vi "read write basic.vi"() -> ()   [LabVIEW 2021]
uses:
  <vilib>/Utility/file.llb/Read Delimited Spreadsheet (string).vi
  <vilib>/Utility/file.llb/Write Delimited Spreadsheet (string).vi
panel:
  out "Read Data":cluster{"Temp Data":dbl, "Message":string}[](array[cluster])
  in  "Write Data":cluster{"Temp Data":dbl, "Message":string}[](array[cluster])
  in  "Write and Read data":bool
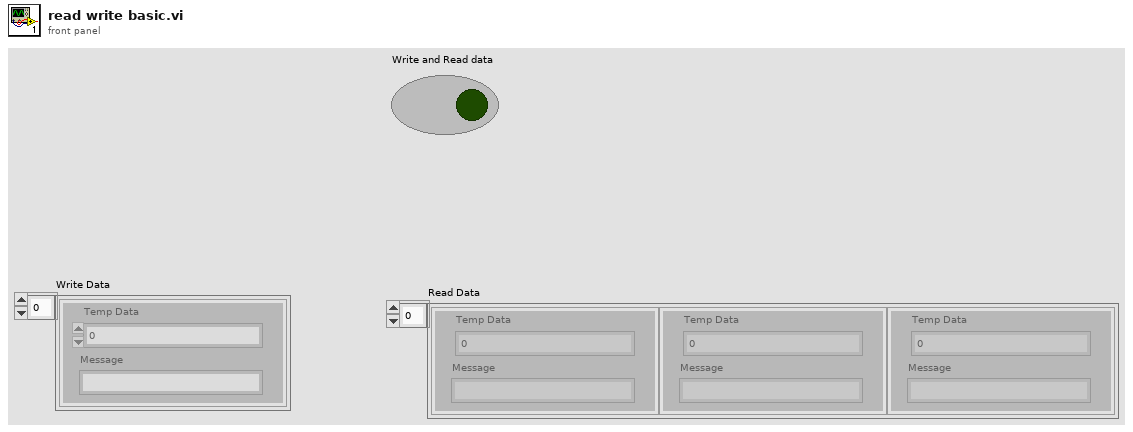
[diagram p1: front panel]
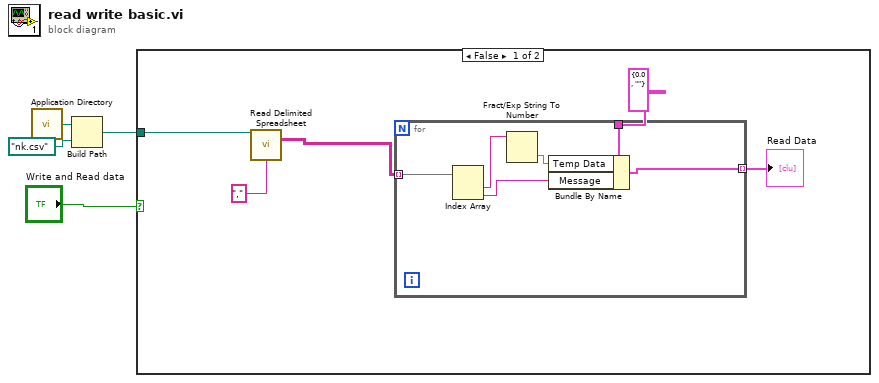
[diagram p0: block diagram]
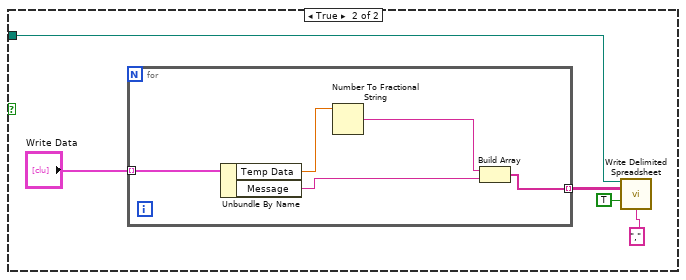
[diagram p2: hidden frame]
diagram:
  n1 = call <vilib>:"Application Directory.vi"() -> ("Application Directory"=w4:path)
  n2 = Build Path(base path=w4, name or relative path=path "nk.csv") -> (appended path=w2:path)
  n3 = case shown="False" "Write and Read data" {
    tunnel: w2 -> [w9 w18]
    frame False {
      n4 = call-poly <vilib>:"Read Delimited Spreadsheet.vi"("file path (dialog if empty)"=w9, "delimiter (\\t)"="," ("delimiter (\\t)")) -> ("all rows"=w5:string[][])  [unwired: 8 in, 5 out]
      n5 = for {
        tunnel: cluster{"Temp Data":dbl, "Message":string} {"Temp Data"=0.0, "Message"=""} ("Cluster") -> [w15]
        tunnel: w5 -> [w11] mode=indexing
        tunnel: [w10] -> w6 mode=indexing
        n6 = Index Array(array=w11) -> (element #1=w13:string, element #2=w14:string)  [unwired: 2 in]
        n7 = Fract/Exp String To Number(string=w13) -> (number=w12:dbl)  [unwired: 3 in, 1 out]
        n8 = Bundle By Name(cluster=w15, "Temp Data"=w12, "Message"=w14) -> (w10:cluster{"Temp Data":dbl, "Message":string})
      }
      "Read Data" <- w6
    }
    frame True {
      n9 = for {
        tunnel: "Write Data" -> [w25] mode=indexing
        tunnel: [w21] -> w16 mode=indexing
        n10 = Unbundle By Name(w25) -> ("Temp Data"=w24:dbl, "Message"=w23:string)
        n11 = Number To Fractional String(number=w24) -> (F-format string=w22:string)  [unwired: 3 in]
        n12 = Build Array(w22, w23) -> (w21:string[])
      }
      n13 = call-poly <vilib>:"Write Delimited Spreadsheet.vi"("file path (dialog if empty)"=w18, "2D data"=w16, "append to file? (new file:F)"=TRUE, "delimiter (\\t)"="," ("delimiter (\\t)")) -> ()  [unwired: 10 in, 2 out]
    }
  }
